vi "UPLOAD LOGIC.vi"(9 "Quantity day":i32[](array[numeric]), 10 "Recipe Names INDEX":i32[](array[numeric]), 11 "TIME DATA":i32[](array[numeric])) -> (3 "PLC DATA":i32[](array[numeric]))   [LabVIEW 2017]
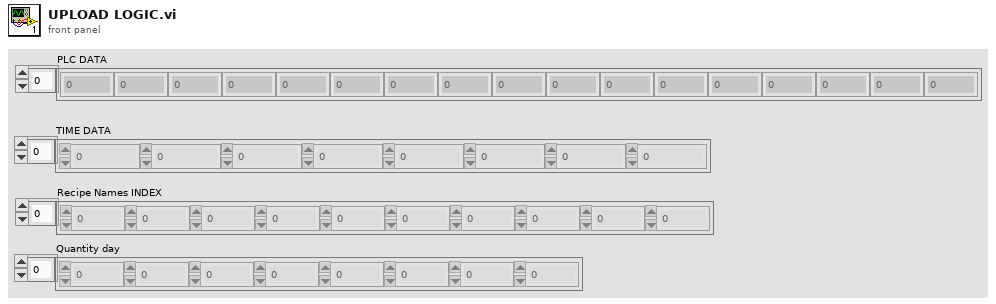
[diagram p1: front panel]
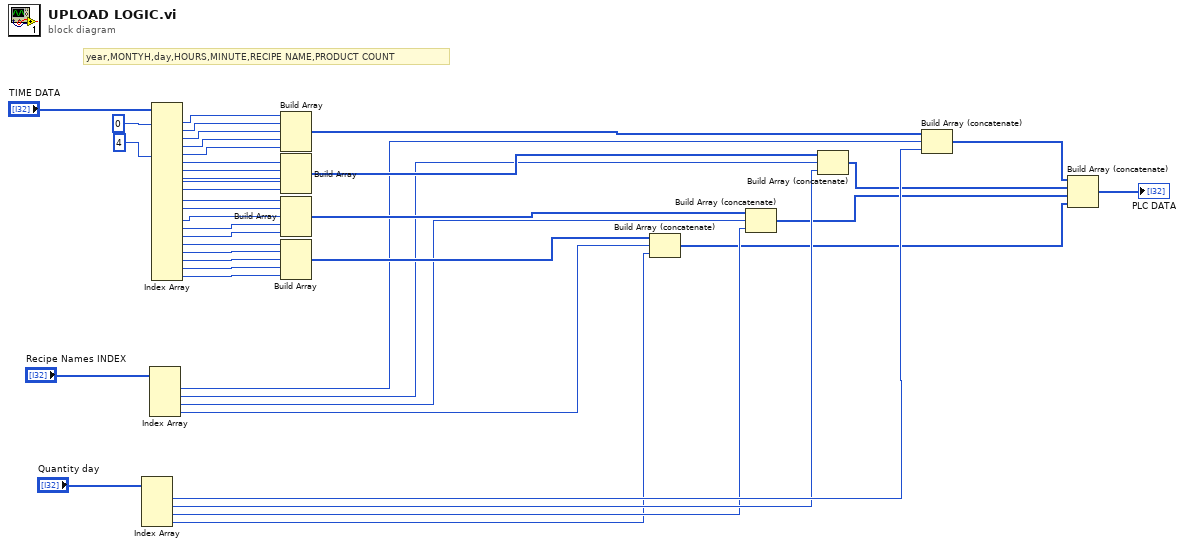
[diagram p0: block diagram]
diagram:
  # "year,MONTYH,day,HOURS,MINUTE,RECIPE NAME,PRODUCT COUNT"
  n1 = Index Array(array="Quantity day") -> (element #1=w33:i32, element #2=w31:i32, element #3=w30:i32, element #4=w29:i32)  [unwired: 4 in]
  n2 = Index Array(array="Recipe Names INDEX") -> (element #1=w27:i32, element #2=w26:i32, element #3=w25:i32, element #4=w24:i32)  [unwired: 4 in]
  n3 = Index Array(array="TIME DATA", index #1=0 ("index"), index #5=4 ("index")) -> (element #1=w39:i32, element #2=w38:i32, element #3=w18:i32, element #4=w17:i32, element #5=w16:i32, element #6=w15:i32, element #7=w14:i32, element #8=w13:i32, element #9=w12:i32, element #10=w11:i32, element #11=w10:i32, element #12=w9:i32, element #13=w8:i32, element #14=w7:i32, element #15=w6:i32, element #16=w5:i32, element #17=w4:i32, element #18=w3:i32, element #19=w2:i32, element #20=w1:i32)  [unwired: 18 in]
  n4 = Build Array(w39, w38, w18, w17, w16) -> (w37:i32[])
  n5 = Build Array(w15, w14, w13, w12, w11) -> (w34:i32[])
  n6 = Build Array(w10, w9, w8, w7, w6) -> (w35:i32[])
  n7 = Build Array(w5, w4, w3, w2, w1) -> (w36:i32[])
  n8 = Build Array (concatenate)(w36, w24, w29) -> (w20:i32[])
  n9 = Build Array (concatenate)(w35, w25, w30) -> (w21:i32[])
  n10 = Build Array (concatenate)(w34, w26, w31) -> (w22:i32[])
  n11 = Build Array (concatenate)(w37, w27, w33) -> (w23:i32[])
  n12 = Build Array (concatenate)(w23, w22, w21, w20) -> (→"PLC DATA":i32[])
